vi "Sandbox.vi"() -> ()   [LabVIEW 2026]
doc: "Sandbox"
panel:
  in  "e":dbl
  out "Result":dbl
  in  "d":dbl
  in  "c":dbl
  in  "b":dbl
  in  "a":dbl
  out "No. Of Iterations Executed - Loop 2":i32
  out "Output - Loop 2":dbl[](array[numeric]) format="%.3f"
  out "No. Of Iterations Executed - Loop 1":i32
  out "Output - Loop 1":dbl[](array[numeric]) format="%.3f"
  out "Stop VI?":bool
  # "Sandbox"
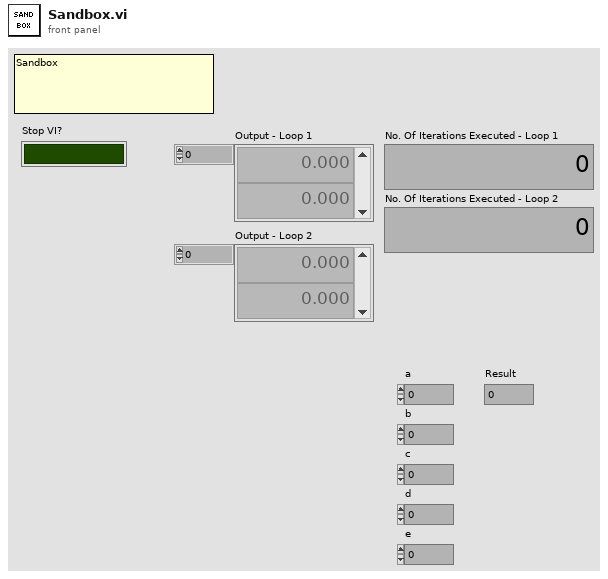
[diagram p1: front panel]
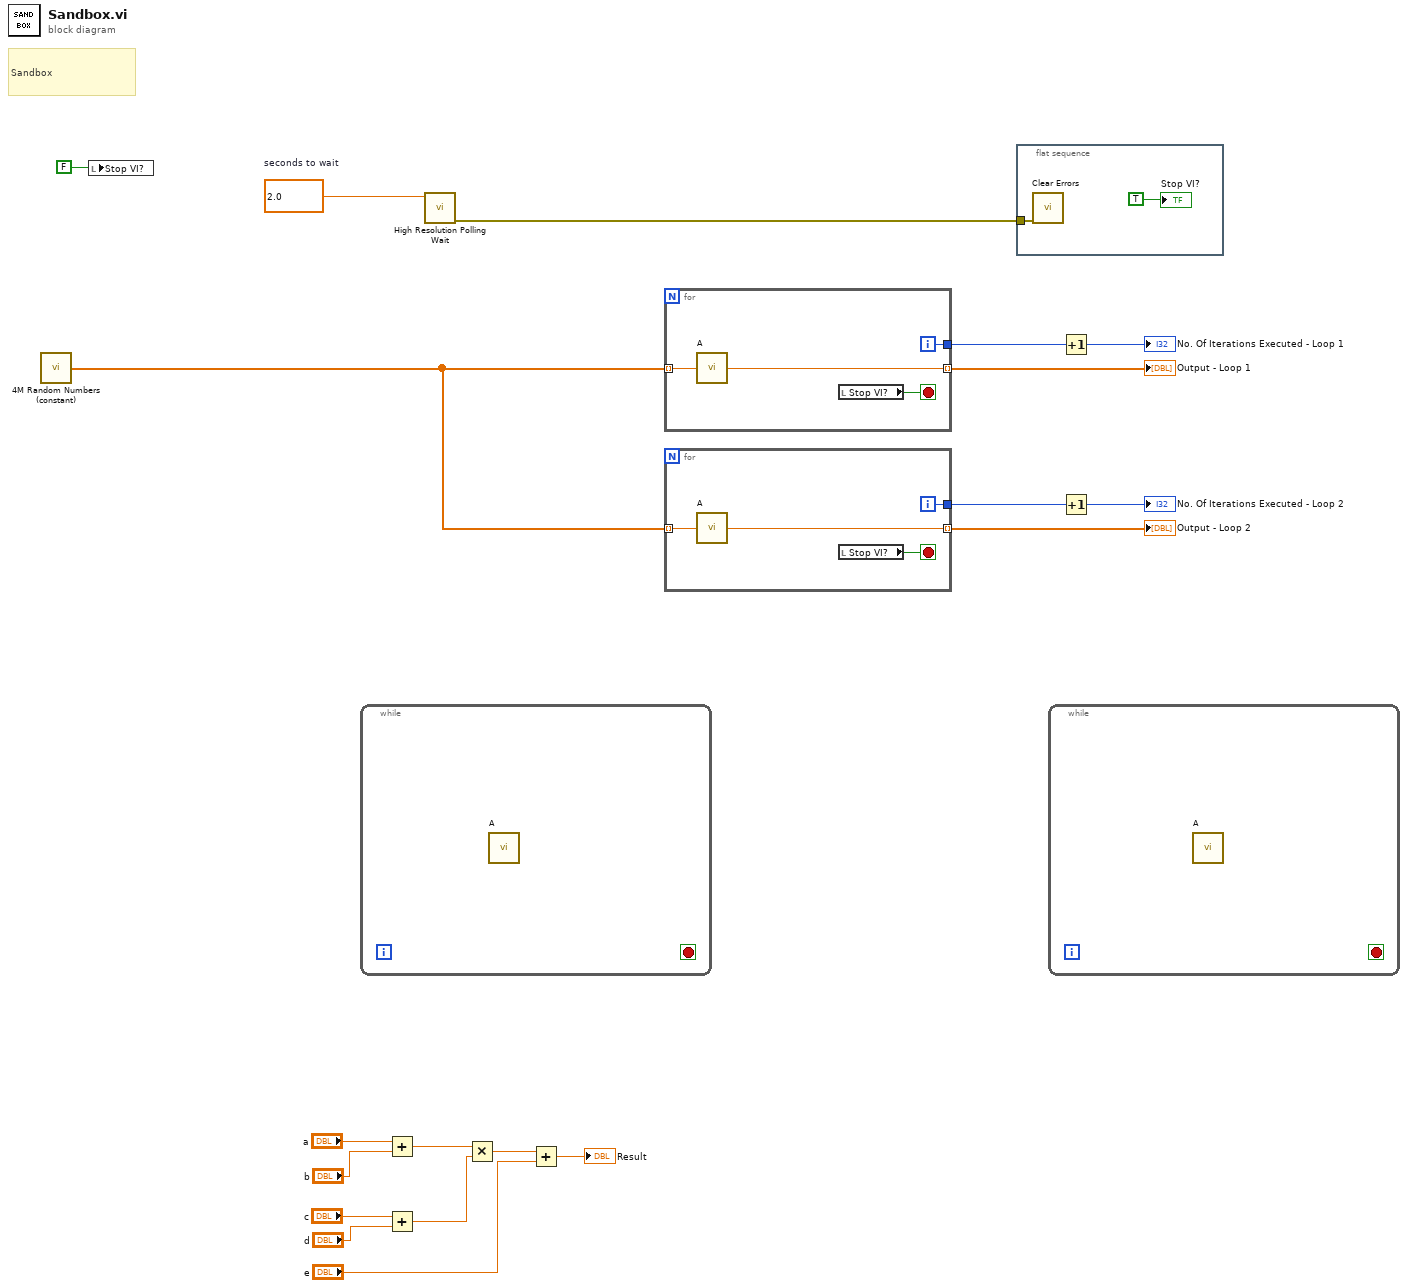
[diagram p0: block diagram]
diagram:
  w13 = 2.0  # seconds to wait
  # "Sandbox"
  n1 = call "4M Random Numbers (constant).vi"() -> ("4M Random Numbers"=w15:dbl[])
  n2 = local write "Stop VI?"(FALSE) -> ()
  n3 = while {
    stop <- _ stop-if-true
    n4 = call "A.vi"() -> ()  [unwired: 1 in, 1 out]
  }
  n5 = Add(x="a", y="b") -> (x+y=w5:dbl)
  n6 = Add(x="c", y="d") -> (x+y=w4:dbl)
  n7 = call <vilib>:"High Resolution Polling Wait.vi"("seconds to wait"=w13) -> ("error out"=w12:errorcluster)  [unwired: 10 in]
  n8 = Multiply(x=w5, y=w4) -> (x*y=w3:dbl)
  n9 = Add(x=w3, y="e") -> (x+y=→"Result":dbl)
  n10 = for {
    tunnel: w15 -> [w23] mode=indexing
    tunnel: [w20] -> w19 mode=indexing
    tunnel: [w21] -> w11
    i -> [w21]
    stop <- w22 stop-if-true
    n11 = call "A.vi"("Input"=w23) -> ("Output"=w20:dbl)
    n12 = local read "Stop VI?"() -> (w22:bool)
  }
  "Output - Loop 1" <- w19
  n13 = for {
    tunnel: w15 -> [w25] mode=indexing
    tunnel: [w24] -> w16 mode=indexing
    tunnel: [w26] -> w10
    i -> [w26]
    stop <- w27 stop-if-true
    n14 = call "A.vi"("Input"=w25) -> ("Output"=w24:dbl)
    n15 = local read "Stop VI?"() -> (w27:bool)
  }
  "Output - Loop 2" <- w16
  n16 = flat-sequence {
    tunnel: w12 -> [w28]
    frame #0 {
      n17 = call <vilib>:"Clear Errors.vi"("error in (no error)"=w28) -> ()  [unwired: 5 in, 2 out]
      "Stop VI?" <- TRUE
    }
  }
  n18 = while {
    stop <- _ stop-if-true
    n19 = call "A.vi"() -> ()  [unwired: 1 in, 1 out]
  }
  n20 = Increment(x=w11) -> (x+1=→"No. Of Iterations Executed - Loop 1":i32)
  n21 = Increment(x=w10) -> (x+1=→"No. Of Iterations Executed - Loop 2":i32)
